vi "supported actions list error handler.vi"(8 "error in (no error)":errorcluster, 11 "Path":path) -> ()   [LabVIEW 2014, in "Simple Sequencer TBM editor node.lvclass"]
doc: "Displays a dialog if there was an issue with the selected Supported Actions List VI."
uses:
  Simple Sequencer TBM editor node.lvclass
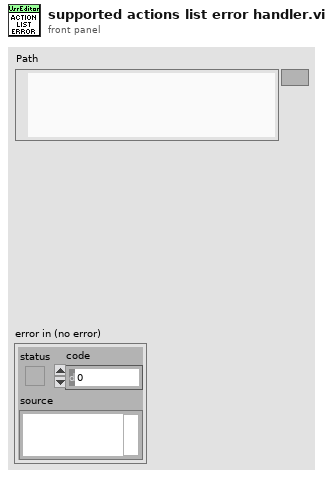
[diagram p1: front panel]
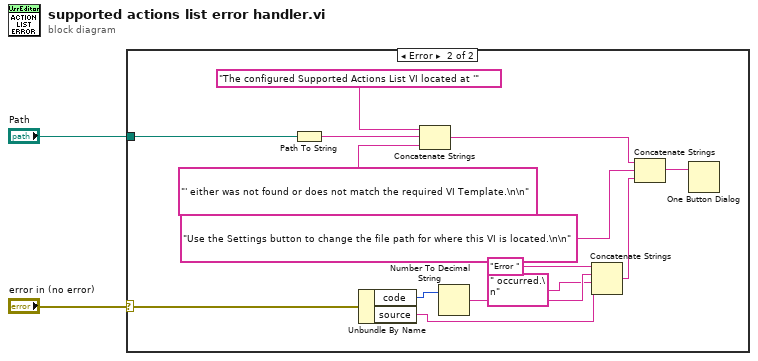
[diagram p0: block diagram]
diagram:
  n1 = case shown="Error" "error in (no error)" {
    selector: "error in (no error)" -> [_ w11]
    tunnel: "Path" -> [_ w12]
    frame No Error {
    }
    frame Error {
      n2 = Path To String(path=w12) -> (string=w14:string)
      n3 = Unbundle By Name(w11) -> ("code"=w16:i32, "source"=w7:string)
      n4 = Concatenate Strings("The configured Supported Actions List VI located at '" ("message"), w14, "' either was not found or does not match the required VI Template.\n\n" ("string")) -> (w5:string)
      n5 = Number To Decimal String(number=w16) -> (decimal integer string=w9:string)  [unwired: 1 in]
      n6 = Concatenate Strings("Error " ("string"), w9, " occurred.\n" ("string"), w7) -> (w4:string)
      n7 = Concatenate Strings(w5, "Use the Settings button to change the file path for where this VI is located.\n\n" ("string"), w4) -> (w6:string)
      n8 = One Button Dialog(message=w6) -> ()  [unwired: 1 in, 1 out]
    }
  }
